vi "圆周长.vi"(11 "Radious":dbl) -> (3 "C":dbl=nan)   [LabVIEW 2012]
doc: "功能：\n\n计算圆形的周长。\n\n公式：\n\nC=2*PI*r"
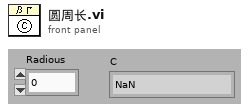
[diagram p1: front panel]
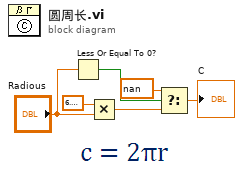
[diagram p0: block diagram]
diagram:
  n1 = Less Or Equal To 0?(x="Radious") -> (x <= 0?=w6:bool)
  n2 = Multiply(x=6.283185307179586, y="Radious") -> (x*y=w2:dbl)
  n3 = Select(t=nan, s=w6, f=w2) -> (s? t:f=→"C":dbl)
